vi "矩阵.vi"() -> ()   [LabVIEW 2010]
doc: "The following example shows the fundamental behavior and functionality of the matrix data type. While the test is running, you can change the matrix inputs or select built-in or user-defined numeric operations. Change the operation mode between matrix and array versions of the operations to see the difference in results."
uses:
  <vilib>/Analysis/Matrix/Numeric/Conversions/Array To Matrix - RA2.vi
  <vilib>/Analysis/Matrix/Numeric/Multiply/Multiply - RM,RM.vi
  <vilib>/Analysis/Matrix/Numeric/Conversions/Matrix To Array - RM.vi
  <vilib>/Analysis/Matrix/NI_Matrix.lvlib
panel:
  in  "数组A":dbl[][](array[numeric])=[[1.0, 0.0], [1.0, 1.0]]
  in  "数组B":dbl[][](array[numeric])=[[1.0, 2.0], [3.0, 4.0]]
  out "矩阵结果":dbl[][](array[numeric])
  out "数组结果":dbl[][](array[numeric])
  in  "数组B":dbl[][](array[numeric])=[[1.0, 2.0], [3.0, 4.0]]
  in  "数组A":dbl[][](array[numeric])=[[1.0, 0.0], [1.0, 1.0]]
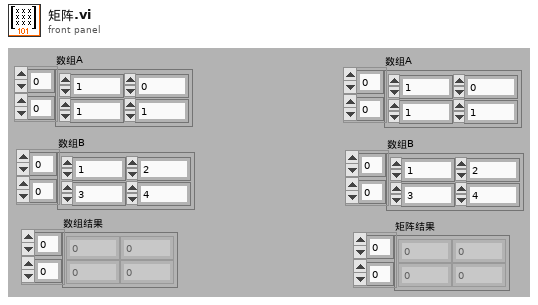
[diagram p1: front panel]
types:
  T1 = typedef "NI_Matrix.lvlib/RealMatrix.ctl" = dbl[][]
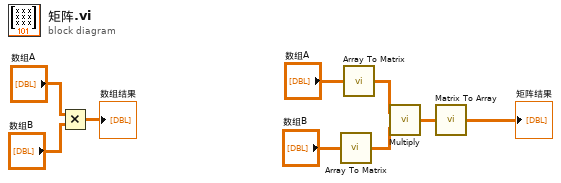
[diagram p0: block diagram]
diagram:
  n1 = Multiply(x="数组A", y="数组B") -> (x*y=→"数组结果":dbl[][])
  n2 = call-poly <vilib>:"Array To Matrix.vi"("Real 2D Array"="数组B") -> ("Real Matrix"=w2:T1)
  n3 = call-poly <vilib>:"Array To Matrix.vi"("Real 2D Array"="数组A") -> ("Real Matrix"=w1:T1)
  n4 = call-poly <vilib>:"Multiply.vi"("Real Matrix B"=w2, "Real Matrix A"=w1) -> ("A * B"=w3:T1)
  n5 = call-poly <vilib>:"Matrix To Array.vi"("Real Matrix"=w3) -> ("Real 2D Array"=→"矩阵结果":dbl[][])
